vi "save FineMask.vi"(8 "Selected Index":dbl[](array[numeric]), 9 "RawData Save Path":path=path "C:/Users/Flash/Desktop/Data/Detector test data", 10 "Text Add":string, 11 "Mask File Raw":path=path "C:/Users/Flash/Desktop/Mask Files/SL066 Detector/SL066_D5_20_align on D3000.csv") -> (3 "Output path":path)   [LabVIEW 2012]
uses:
  <vilib>/Utility/file.llb/Read From Spreadsheet File (string).vi
  <vilib>/Utility/file.llb/Write To Spreadsheet File (string).vi
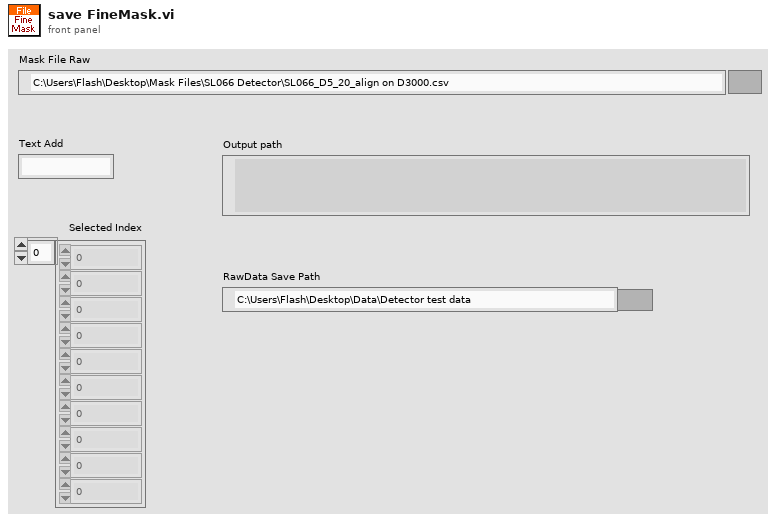
[diagram p1: front panel]
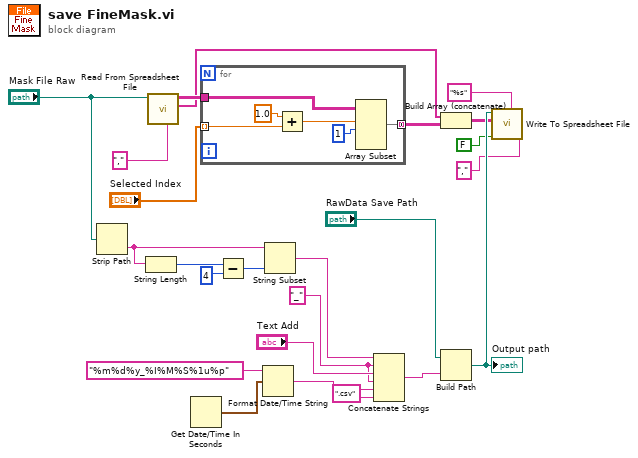
[diagram p0: block diagram]
diagram:
  w2 = "_" ("string")
  n1 = Strip Path(path="Mask File Raw") -> (name=w24:string)  [unwired: 1 out]
  n2 = String Length(string=w24) -> (length=w23:i32)
  n3 = call-poly <vilib>:"Read From Spreadsheet File.vi"("delimiter (\\t)"="," ("delimiter (\\t)"), "file path (dialog if empty)"="Mask File Raw") -> ("first row"=w14:string[], "all rows"=w16:string[][])  [unwired: 5 in, 3 out]
  n4 = Get Date/Time In Seconds() -> (seconds since 1Jan1904=w1:timestamp)
  n5 = for {
    tunnel: "Selected Index" -> [w27] mode=indexing
    tunnel: w16 -> [w30]
    tunnel: [w28] -> w13 mode=concatenating
    n6 = Add(x=1.0, y=w27) -> (x+y=w25:dbl)
    n7 = Array Subset(array=w30, index (row)=w25, length (row)=1 ("length")) -> (w28:string[][])  [unwired: 2 in]
  }
  n8 = Subtract(x=w23, y=4) -> (x-y=w21:i32)
  n9 = Format Date/Time String(time format string (%c)="%m%d%y_%I%M%S%1u%p", seconds (now)=w1) -> (date/time string=w4:string)  [unwired: 1 in]
  n10 = String Subset(string=w24, length (rest)=w21) -> (substring=w3:string)  [unwired: 1 in]
  n11 = Concatenate Strings(w3, w2, "Text Add", w2, w4, ".csv" ("string")) -> (w19:string)
  n12 = Build Array (concatenate)(w14, w13) -> (w10:string[][])
  n13 = Build Path(base path="RawData Save Path", name or relative path=w19) -> (appended path=w11:path)
  "Output path" <- w11
  n14 = call-poly <vilib>:"Write To Spreadsheet File.vi"("delimiter (\\t)"="," ("delimiter (\\t)"), "format (%s)"="%s" ("format (%.3f)"), "append to file? (new file:F)"=FALSE, "2D data"=w10, "file path (dialog if empty)"=w11) -> ()  [unwired: 3 in, 1 out]
